vi "Agilent DMM Read Calibration Status.vi"(7 "Agilent DMM":T1, 8 "error in (no error)":errorcluster, 11 "VISA Resource Name":refnum<visa-resource-name>) -> (0 "error out":errorcluster {"code" format="%.0x"}, 1 "Null Value":dbl, 2 "Calibrated?":bool, 3 "dup VISA Resource Name":refnum<visa-resource-name>)   [LabVIEW 2011]
uses:
  TypeDefs/Agilent DMM Instrument Info.ctl
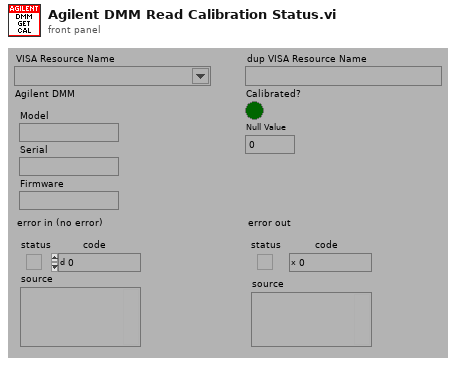
[diagram p1: front panel]
types:
  T1 = typedef "Agilent DMM Instrument Info.ctl" = cluster{"Model":string, "Serial":string, "Firmware":string}
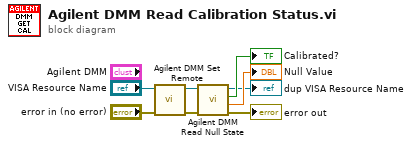
[diagram p0: block diagram]
diagram:
  n1 = call "Agilent DMM Set Remote.vi"("error in (no error)"="error in (no error)", "VISA Resource Name"="VISA Resource Name") -> ("error out"=w5:errorcluster, "dup VISA Resource Name"=w6:refnum<visa-resource-name>)  [unwired: 8 out]
  n2 = call "Agilent DMM Read Null State.vi"("error in (no error)"=w5, "VISA Resource Name"=w6) -> ("error out"=→"error out":errorcluster, "Null Value"=→"Null Value":dbl, "Calibrated?"=→"Calibrated?":bool, "dup VISA Resource Name"=→"dup VISA Resource Name":refnum<visa-resource-name>)  [unwired: 6 out]
